vi "SpeedAccelDeccelPositionM2.vi"(4 "Position":i32 max=127 step=1, 5 "Deccel":u32 max=127 step=1, 6 "Immediate":u8 max=127 step=1, 7 "Accel":u32 max=127 step=1, 8 "error in (no error)":errorcluster, 9 "Address":u8, 10 "Speed":u32 max=127 step=1, 11 "VISA Refnum in":refnum<visa-resource-name>) -> (0 "error out":errorcluster, 2 "Valid":bool, 3 "VISA Refnum out":refnum<visa-resource-name>)   [LabVIEW 2015, in "Ion Motion Roboclaw.lvlib"]
uses:
  <instrlib>/Ion Motion Roboclaw/Ion Motion Roboclaw.lvlib
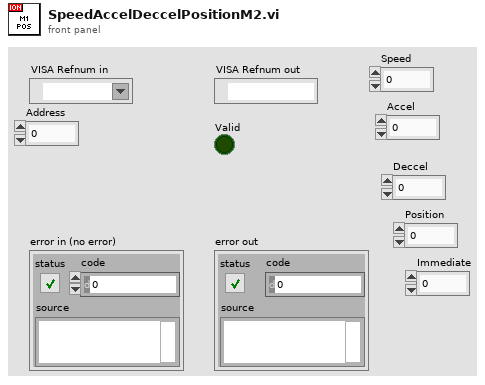
[diagram p1: front panel]
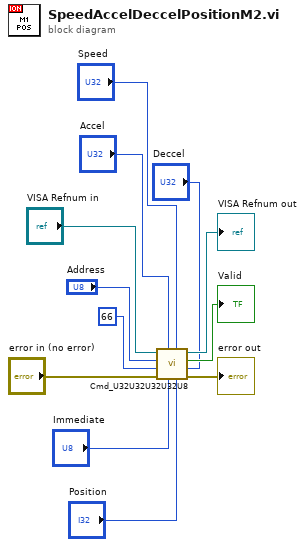
[diagram p0: block diagram]
diagram:
  n1 = call <instrlib>:"Cmd_U32U32U32U32U8.vi"("Arg3"="Deccel", "Arg4"="Position", "Arg2"="Speed", "Arg5"="Immediate", "Arg1"="Accel", "error in (no error)"="error in (no error)", "Cmd"=u8 66, "Address"="Address", "VISA Refnum in"="VISA Refnum in") -> ("error out"=→"error out":errorcluster, "Valid"=→"Valid":bool, "VISA Refnum out"=→"VISA Refnum out":refnum<visa-resource-name>)
